vi "Day 19-Compute Linear Offset.vi"(9 "Rotation":T1, 10 "Reference Known Beacon":i32[](array[numeric]), 11 "Current Beacon Compare Point":i32[](array[numeric])) -> (3 "Offset":i32[](array[numeric]))   [LabVIEW 2021]
uses:
  <vilib>/Analysis/Matrix/Datatypes/RealMatrix.ctl
  <vilib>/Analysis/Matrix/Numeric/Multiply/Multiply - RM,RM.vi
  <vilib>/Analysis/Matrix/Numeric/Conversions/Matrix To Array - RM.vi
  <vilib>/Analysis/Matrix/NI_Matrix.lvlib
  <vilib>/Analysis/Matrix/Numeric/Conversions/Array To Matrix - RA.vi
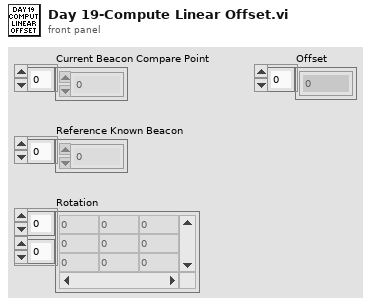
[diagram p1: front panel]
types:
  T1 = typedef "NI_Matrix.lvlib/RealMatrix.ctl" = dbl[][]
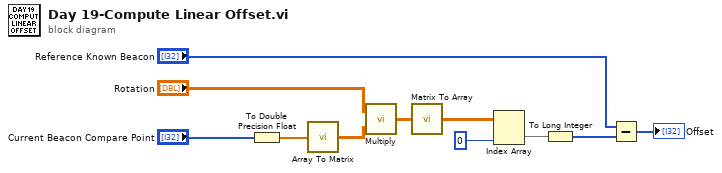
[diagram p0: block diagram]
diagram:
  n1 = To Double Precision Float(number="Current Beacon Compare Point") -> (double precision float=w2:dbl[])
  n2 = call-poly <vilib>:"Array To Matrix.vi"("Real 1D Array"=w2) -> ("Real Matrix (Column Vector)"=w9:T1)
  n3 = call-poly <vilib>:"Multiply.vi"("Real Matrix B"=w9, "Real Matrix A"="Rotation") -> ("A * B"=w10:T1)
  n4 = call-poly <vilib>:"Matrix To Array.vi"("Real Matrix"=w10) -> ("Real 2D Array"=w11:dbl[][])
  n5 = Index Array(array=w11, index (col)=0 ("disabled index (col)")) -> (element=w6:dbl[])  [unwired: 1 in]
  n6 = To Long Integer(number=w6) -> (32bit integer=w7:i32[])
  n7 = Subtract(x="Reference Known Beacon", y=w7) -> (x-y=→"Offset":i32[])
